vi "SPU_Sampling_Start.vi"(7 "错误输入（无错误）":errorcluster, 10 "引用":refnum<k24>) -> (0 "error IO":errorcluster, 3 "引用输出":refnum<k24>)   [LabVIEW 2017]
doc: "SPU sampling start"
uses:
  D:/test/ILSTS/LV_IL/LV_IL_Sample_x86/DLL/InstrumentDLL.dll
  DLL/InstrumentDLL.dll
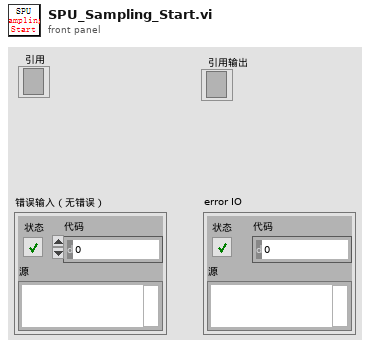
[diagram p1: front panel]
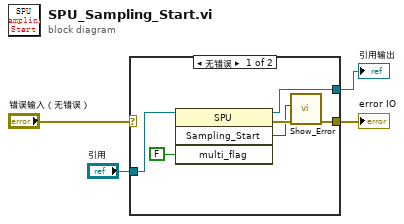
[diagram p0: block diagram]
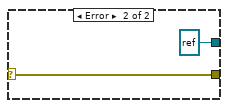
[diagram p2: hidden frame]
diagram:
  n1 = case shown="无错误" "错误输入（无错误）" {
    selector: "错误输入（无错误）" -> [_ w12]
    tunnel: [w8 w12] -> w2
    tunnel: [w7 refnum<k24> refnum ("new reference")] -> w3
    tunnel: "引用" -> [w5 _]
    frame No Error {
      n2 = invoke class="SPU" method="Sampling_Start"(reference=w5, "multi_flag"=FALSE) -> (reference out=w7:refnum<k24>, error out=w10:errorcluster, "Sampling_Start"=w9:i32)  [unwired: 2 in, 1 out]
      n3 = call "Show_Error.vi"("error in (no error)"=w10, "Error"=w9) -> ("error out"=w8:errorcluster)  [unwired: 9 in]
    }
    frame Error {
    }
  }
  "引用输出" <- w3
  "error IO" <- w2
